vi "SaveArrayToTxt.vi"(1 "Input array":dbl[][](array[numeric]), 3 "Filename":string="Trial_sequence", 4 "File path":path=path "D:/Data/trackingresults") -> (0 "Boolean":bool=TRUE)   [LabVIEW 2013]
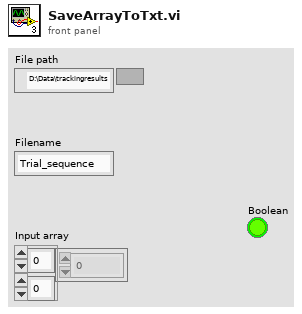
[diagram p1: front panel]
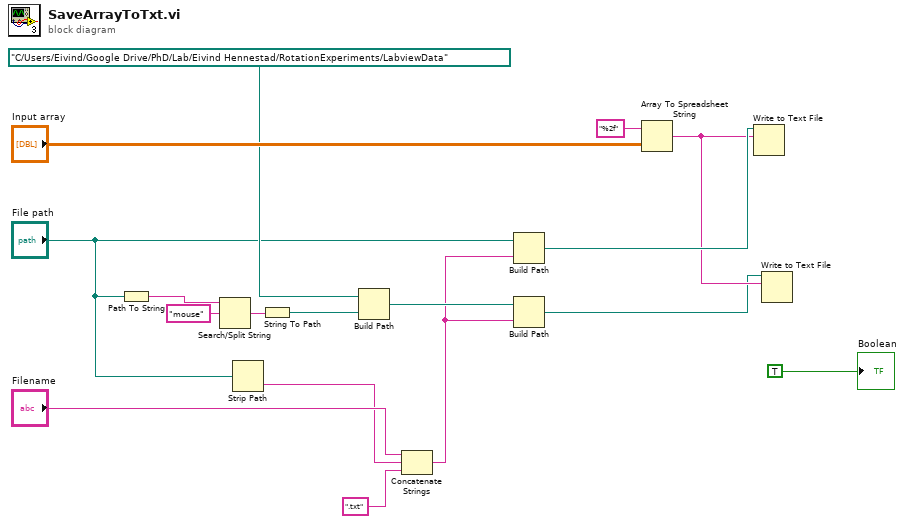
[diagram p0: block diagram]
diagram:
  n1 = Path To String(path="File path") -> (string=w11:string)
  n2 = Search/Split String(string=w11, search string/char (-)="mouse") -> (match + rest of string=w9:string)  [unwired: 1 in, 2 out]
  n3 = Strip Path(path="File path") -> (name=w1:string)  [unwired: 1 out]
  n4 = String To Path(string=w9) -> (path=w7:path)
  n5 = Build Path(base path=path "C:/Users/Eivind/Google Drive/PhD/Lab/Eivind Hennestad/RotationExperiments/LabviewData", name or relative path=w7) -> (appended path=w6:path)
  n6 = Concatenate Strings("Filename", w1, ".txt" ("string")) -> (w5:string)
  n7 = Build Path(base path="File path", name or relative path=w5) -> (appended path=w15:path)
  n8 = Build Path(base path=w6, name or relative path=w5) -> (appended path=w3:path)
  n9 = Array To Spreadsheet String(array="Input array", 3:"%2f" ("format string")) -> (spreadsheet string=w4:string)  [unwired: 1 in]
  n10 = Write to Text File(file (use dialog)=w15, text=w4) -> ()  [unwired: 2 in, 3 out]
  n11 = Write to Text File(file (use dialog)=w3, text=w4) -> ()  [unwired: 2 in, 3 out]
  "Boolean" <- TRUE
